vi "Method_Const.vi"(4 "Value":cxt, 5 "Value A":refnum<class "Abs_Complex Extended Float.lvclass">) -> (1 "Result":refnum<class "Abs_Boolean.lvclass">)   [LabVIEW 2021, in "Not Equal_CPLX_EXT.lvclass"]
uses:
  Not Equal_CPLX_EXT.lvclass
  Abs_Types/Complex Extended Float/Abs_Complex Extended Float.lvclass
  C:/Program Files (x86)/National Instruments/LabVIEW 2021/vi.lib/TSA/Abstract Data Classes/Abs_Types/Numeric/Abs_Numeric.lvclass
  Abs_Types/Boolean/Abs_Boolean.lvclass
  C:/TSA/LV_Abstract/Source/Functions/Support/Compare/Two Term/CPLX_EXT/AbsComp_Two Term_CPLX_EXT.lvclass
  C:/Program Files (x86)/National Instruments/LabVIEW 2021/vi.lib/TSA/Abstract Data Classes/Abs_Types/Boolean/Abs_Boolean.lvclass
  Support/Compare/Two Term/CPLX_EXT/AbsComp_Two Term_CPLX_EXT.lvclass/AbsComp_Two Term_CPLX_EXT.ctl
  Support/Compare/Two Term/CPLX_EXT/Properties/Write Numeric A.vi
  Support/Compare/Two Term/CPLX_EXT/Properties/Write Numeric B.vi
  Constants/Support/CPLX_EXT/Const_CPLX_EXT.lvclass
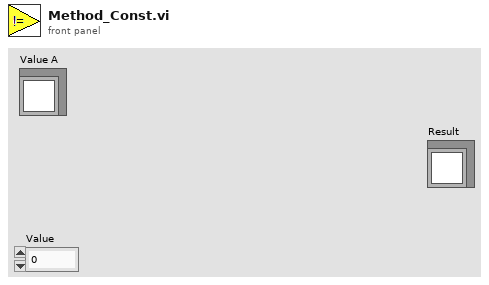
[diagram p1: front panel]
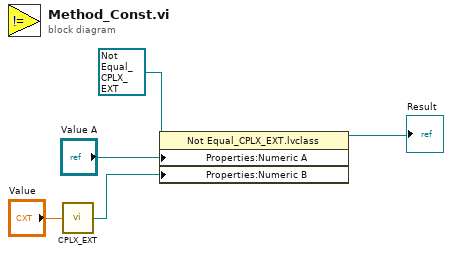
[diagram p0: block diagram]
diagram:
  n1 = call "CPLX_EXT.vi"("Value"="Value") -> ("Constant"=w2:refnum<class "Abs_Complex Extended Float.lvclass">)  [unwired: 4 in]
  n2 = property class="Not Equal_CPLX_EXT.lvclass"(reference=refnum<class "Not Equal_CPLX_EXT.lvclass"> refnum ("Greater 0_U64.lvclass"), "Properties:Numeric A"="Value A", "Properties:Numeric B"=w2) -> (reference out=→"Result":refnum<class "Not Equal_CPLX_EXT.lvclass">)  [unwired: 1 in, 1 out]
